vi "Set SG Path.vi"(0 "Path in":refnum<class "SG Path.lvclass">, 5 "Cal point in":T1, 11 "error in":errorcluster) -> (4 "Path out":refnum<class "SG Path.lvclass">, 6 "Cal point out":T1, 8 "Source Gain":dbl, 10 "Digital Gain":dbl, 15 "error out":errorcluster)   [LabVIEW 2023, in "RFFixtureCharact.RMM.lvlib" / "SG Path.lvclass"]
uses:
  SG Path.lvclass
  Public/Base Classes/Scalar/Scalar Path/Type Definitions/Cal Point.ctl
  Public/Base Classes/Scalar/SG Path/SG Path.lvclass
  SG Path.lvclass/SG Path.ctl
  Public/Base Classes/Scalar/Scalar Path/Scalar Path.lvclass
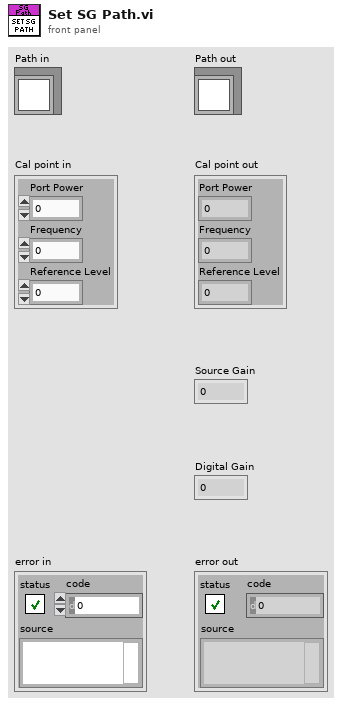
[diagram p1: front panel]
types:
  T1 = typedef "RFFixtureCharact.Public.lvlib/Scalar Path.lvclass/Cal Point.ctl" = cluster{"Port Power":dbl, "Frequency":dbl, "Reference Level":dbl}
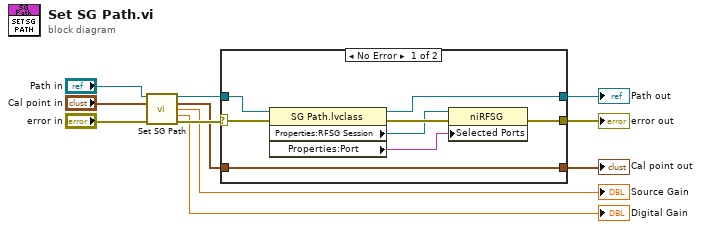
[diagram p0: block diagram]
diagram:
  n1 = call-parent "Set SG Path.vi"("Path in"="Path in", "Cal point in"="Cal point in", "error in (no error)"="error in") -> ("Path out"=w7:refnum<class "SG Path.lvclass">, "Cal point out"=w6:T1, "Source Gain"=→"Source Gain":dbl, "Digital Gain"=→"Digital Gain":dbl, "error out"=w8:errorcluster)  [unwired: 8 in]
  n2 = case shown="No Error" w8 {
    selector: w8 -> [w19 w22]
    tunnel: w7 -> [w18 w21]
    tunnel: [w15 w21] -> w4
    tunnel: [w14 w22] -> w5
    tunnel: [w13 w20] -> w3
    tunnel: w6 -> [w13 w20]
    frame No Error {
      n3 = property class="SG Path.lvclass"(reference=w18, error in=w19) -> (reference out=w15:refnum<class "SG Path.lvclass">, error out=w17:errorcluster, "Properties:RFSG Session"=w16:refnum<k15>, "Properties:Port"=w12:string)
      n4 = property class="niRFSG"(reference=w16, error in=w17, "Selected Ports"=w12) -> (error out=w14:errorcluster)  [unwired: 1 out]
    }
    frame Error {
    }
  }
  "error out" <- w5
  "Cal point out" <- w3
  "Path out" <- w4
